vi "MACBIN Open File Refnum__ogtk.vi"(4 "resource fork (F)":bool, 5 "error in (no error)":errorcluster, 6 "deny mode (2)":T1(ring)=enum."deny none", 7 "open mode (0)":T2(ring), 8 "file path":path) -> (0 "error out":errorcluster, 3 "file refnum":refnum<file>)   [LabVIEW 2014]
uses:
  <userlib>/_OpenG.lib/lvzip/lvzlib.dll
panel:
  in  "dummy refnum":refnum<file>
  # "Please visit http://www.OpenG.org to learn about the\nOpen Source LabVIEW software movement.\n\nNOTICE -- YOU MUST LEAVE THIS NOTICE IN PLACE.  PER THE TERMS OF THE LICENSE BELOW, YOU MAY SUBLICENSE THIS SOFTWARE \nIN ANY WAY THAT DOES NOT CONFLICT WITH THIS LICENSE.\n\n### BSD License (http://www.opensource.org/licenses/bsd-license.php) Begin ###\n \nCopyright (C) 2002 Christophe Salzmann christophe.salzmann@epfl.ch\nCopyright (C) 2002-2006 Rolf Kalbermatter rolf.kalbermatter@citengineering.com\n\nAll rights reserved.\n\nRedistribution and use in source and binary forms, with or without modification, are permitted provided that the following conditions are met:\n\n    * Redistributions of source code must retain the above copyright notice, this list of conditions and the following disclaimer.\n    * Redistributions in binary form must reproduce the above copyright notice, this list of conditions and the following disclaimer in the \n       documentation and/or other materials provided with the distribution.\n    * Neither the name of SciWare, James Kring, Inc., nor the names of its contributors may be used to endorse or promote products derived \n       from this software without specific prior written permission.\n\nTHIS SOFTWARE IS PROVIDED BY THE COPYRIGHT HOLDERS AND CONTRIBUTORS \"AS IS\" AND ANY EXPRESS OR IMPLIED WARRANTIES, \nINCLUDING, BUT NOT LIMITED TO, THE IMPLIED WARRANTIES OF MERCHANTABILITY AND FITNESS FOR A PARTICULAR PURPOSE ARE \nDISCLAIMED. IN NO EVENT SHALL THE COPYRIGHT OWNER OR CONTRIBUTORS BE LIABLE FOR ANY DIRECT, INDIRECT, INCIDENTAL,\n SPECIAL, EXEMPLARY, OR CONSEQUENTIAL DAMAGES (INCLUDING, BUT NOT LIMITED TO, PROCUREMENT OF SUBSTITUTE GOODS OR \nSERVICES; LOSS OF USE, DATA, OR PROFITS; OR BUSINESS INTERRUPTION) HOWEVER CAUSED AND ON ANY THEORY OF LIABILITY, \nWHETHER IN CONTRACT, STRICT LIABILITY, OR TORT (INCLUDING NEGLIGENCE OR OTHERWISE) ARISING IN ANY WAY OUT OF THE USE \nOF THIS SOFTWARE, EVEN IF ADVISED OF THE POSSIBILITY OF SUCH DAMAGE.\n\n### BSD License End ###"
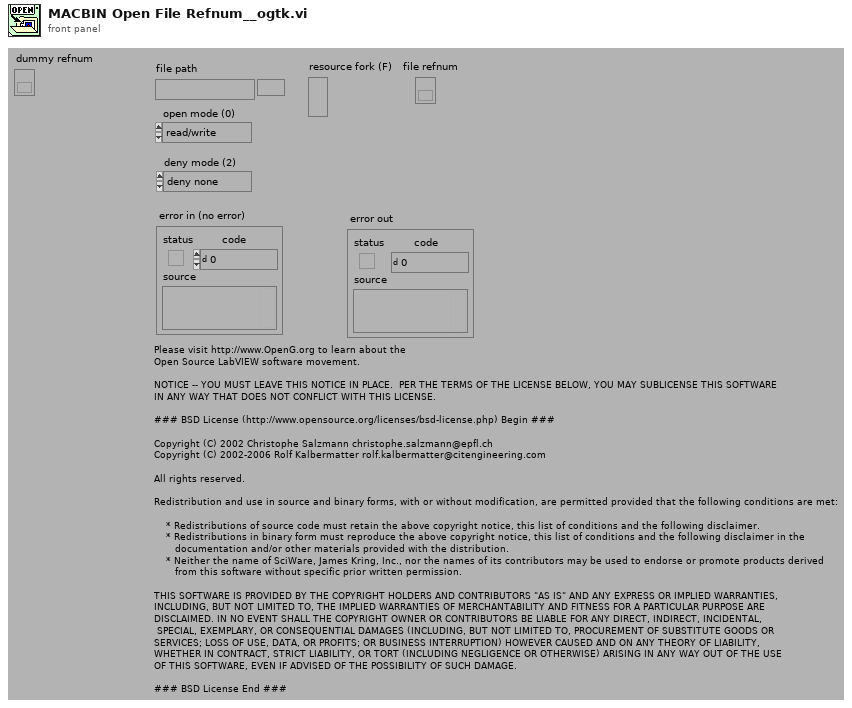
[diagram p1: front panel]
types:
  T1 = enum16{"deny read/write", "deny write-only", "deny none"}
  T2 = enum16{"read/write", "read-only", "write-only", "write-only (truncate)"}
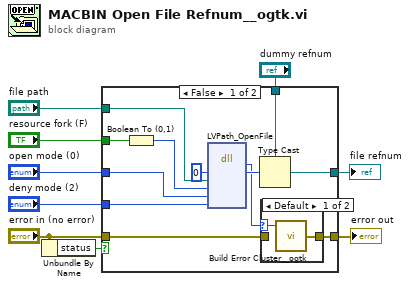
[diagram p0: block diagram]
diagram:
  n1 = Unbundle By Name("error in (no error)") -> ("status"=w8:bool)
  n2 = case shown="False" w8 {
    tunnel: "file path" -> [w18 _]
    tunnel: "error in (no error)" -> [w21 w26]
    tunnel: [w13 w25] -> w6
    tunnel: "open mode (0)" -> [w16 _]
    tunnel: [w20 w26] -> w4
    tunnel: "deny mode (2)" -> [w17 _]
    tunnel: "dummy refnum" -> [w14 w25]
    tunnel: "resource fork (F)" -> [w11 _]
    frame False {
      n3 = Boolean To (0,1)(Boolean=w11) -> (0, 1=w10:i16)
      n4 = dll-call lib="C:/Program Files/National Instruments/LabVIEW 2014/user.lib/_OpenG.lib/lvzip/lvzlib.*" fn="LVPath_OpenFile"("refnum"=u32 0, "file path"=w18, "rsrc"=w10, "openMode"=w16, "denyMode"=w17) -> (w12:i32, "refnum"=w15:u32)  [unwired: 7 in, 2 out]
      n5 = Type Cast(type=w14, x=w15) -> (*(type *) &x=w13:refnum<file>)
      n6 = case shown="Default" w12 {
        selector: w12 -> [w23 _]
        tunnel: w21 -> [_ w24]
        tunnel: [w22 w24] -> w20
        frame Default {
          n7 = call "Build Error Cluster__ogtk.vi"("code"=w23) -> ("error out"=w22:errorcluster)  [unwired: 1 in]
        }
        frame 0 {
        }
      }
    }
    frame True {
    }
  }
  "error out" <- w4
  "file refnum" <- w6
